vi "CRC16 (子VI).vi"(11 "字符串":string) -> (3 "数值":u16)   [LabVIEW 2023]
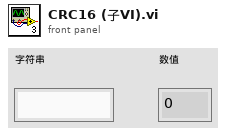
[diagram p1: front panel]
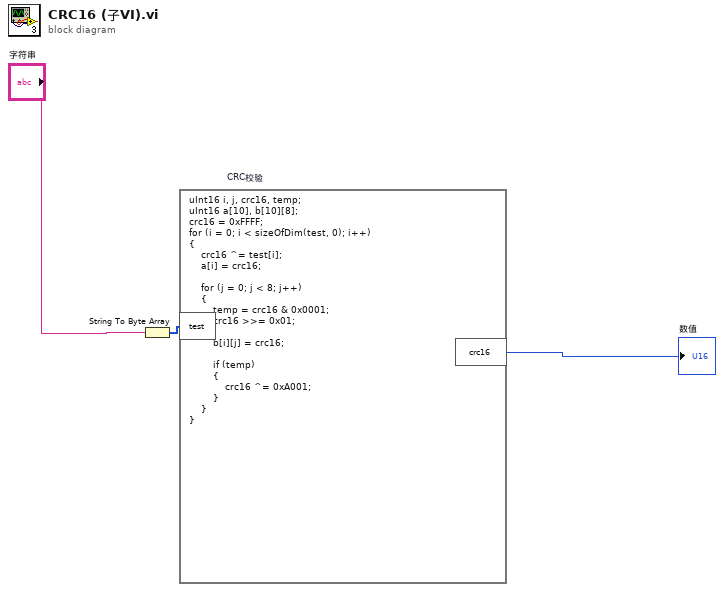
[diagram p0: block diagram]
diagram:
  n1 = String To Byte Array(string="字符串") -> (unsigned byte array=w1:u8[])
  n2 = formula code="uInt16 i, j, crc16, temp;\nuInt16 a[10], b[10][8];\ncrc16 = 0xFFFF;\nfor (i = 0; i < sizeOfDim(test, 0); i++)\n{\n    crc16 ^= test[i];\n    a[i] = crc16;\n\n    for (j = 0; j < 8; j++)\n    {\n        temp = crc16 & 0x0001;\n        crc16 >>= 0x01;\n\n        b[i][j] = crc16;\n\n        if (temp)\n        {\n            crc16 ^= 0xA001;\n        }\n    }\n}" "CRC校验"("test"=w1) -> ("crc16"=→"数值":u16)
